vi "TagLayoutConvert.vi"(0 "Layout":string) -> (1 "Pixel Map":u8[][](array[numeric]), 2 "Size":i32, 3 "Number Of Bits":i32)   [LabVIEW 2020, in "feature_detection.lvlib"]
uses:
  feature_detection.lvlib
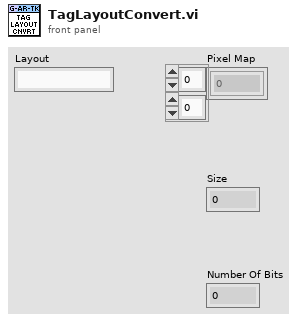
[diagram p1: front panel]
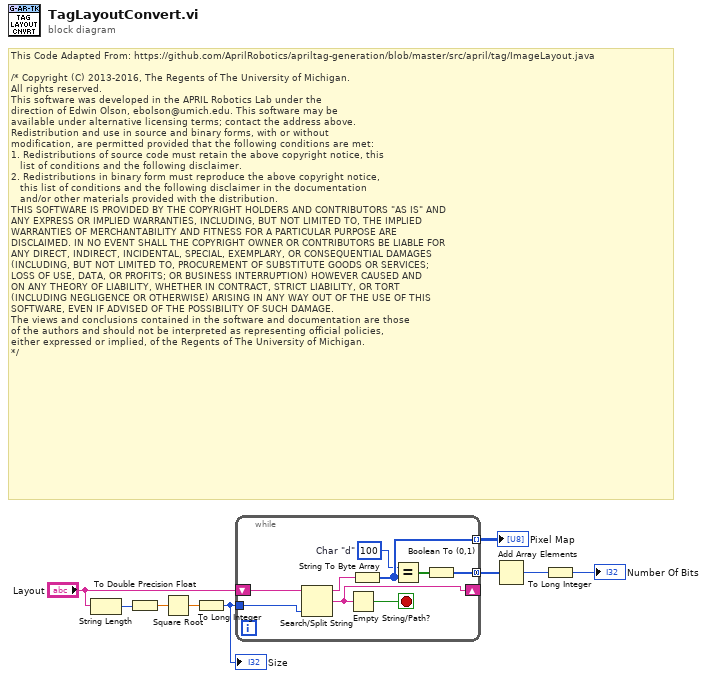
[diagram p0: block diagram]
diagram:
  # "This Code Adapted From: https://github.com/AprilRobotics/apriltag-generation/blob/master/src/april/tag/ImageLayout.java\n\n/* Copyright (C) 2013-2016, The Regents of The University of Michigan.\nAll rights reserved.\nThis software was developed in the APRIL Robotics Lab under the\ndirection of Edwin Olson, ebolson@umich.edu. This software may be\navailable under alternative licensing terms; contact the address above.\nRedistribution and use in source and binary forms, with or without\nmodification, are permitted provided that the following conditions are met:\n1. Redistributions of source code must retain the above copyright notice, this\n   list of conditions and the following disclaimer.\n2. Redistributions in binary form must reproduce the above copyright notice,\n   this list of conditions and the following disclaimer in the documentation\n   and/or other materials provided with the distribution.\nTHIS SOFTWARE IS PROVIDED BY THE COPYRIGHT HOLDERS AND CONTRIBUTORS \"AS IS\" AND\nANY EXPRESS OR IMPLIED WARRANTIES, INCLUDING, BUT NOT LIMITED TO, THE IMPLIED\nWARRANTIES OF MERCHANTABILITY AND FITNESS FOR A PARTICULAR PURPOSE ARE\nDISCLAIMED. IN NO EVENT SHALL THE COPYRIGHT OWNER OR CONTRIBUTORS BE LIABLE FOR\nANY DIRECT, INDIRECT, INCIDENTAL, SPECIAL, EXEMPLARY, OR CONSEQUENTIAL DAMAGES\n(INCLUDING, BUT NOT LIMITED TO, PROCUREMENT OF SUBSTITUTE GOODS OR SERVICES;\nLOSS OF USE, DATA, OR PROFITS; OR BUSINESS INTERRUPTION) HOWEVER CAUSED AND\nON ANY THEORY OF LIABILITY, WHETHER IN CONTRACT, STRICT LIABILITY, OR TORT\n(INCLUDING NEGLIGENCE OR OTHERWISE) ARISING IN ANY WAY OUT OF THE USE OF THIS\nSOFTWARE, EVEN IF ADVISED OF THE POSSIBILITY OF SUCH DAMAGE.\nThe views and conclusions contained in the software and documentation are those\nof the authors and should not be interpreted as representing official policies,\neither expressed or implied, of the Regents of The University of Michigan.\n*/"
  n1 = String Length(string="Layout") -> (length=w2:i32)
  n2 = To Double Precision Float(number=w2) -> (double precision float=w6:dbl)
  n3 = Square Root(x=w6) -> (sqrt(x)=w7:dbl)
  n4 = To Long Integer(number=w7) -> (32bit integer=w3:i32)
  "Size" <- w3
  n5 = while {
    shift-right: [w16] -> _
    shift-left: "Layout" -> [w18]
    tunnel: [w13] -> w1 mode=indexing
    tunnel: w3 -> [w14]
    tunnel: [w10] -> w5 mode=concatenating
    stop <- w15 stop-if-true
    w12 = u8 100  # Char "d"
    n6 = Search/Split String(string=w18, offset (0)=w14) -> (substring before match=w17:string, match + rest of string=w16:string)  [unwired: 1 in, 1 out]
    n7 = Empty String/Path?(string/path=w16) -> (empty?=w15:bool)
    n8 = String To Byte Array(string=w17) -> (unsigned byte array=w13:u8[])
    n9 = Equal?(x=w12, y=w13) -> (x = y?=w11:bool[])
    n10 = Boolean To (0,1)(Boolean=w11) -> (0, 1=w10:i16[])
  }
  "Pixel Map" <- w1
  n11 = Add Array Elements(numeric array=w5) -> (sum=w4:i16)
  n12 = To Long Integer(number=w4) -> (32bit integer=→"Number Of Bits":i32)
